vi "EventLog.Gui.vi"() -> ()   [LabVIEW 2016]
uses:
  <vilib>/Utility/miscctls.llb/LVRowAndColumnUnsignedTypeDef.ctl
  EventLog.Buffer.Action.ctl
  Global/ApplicationGlobal.vi
  Config/Config.Global.vi
  Translator/Translator.Global.vi
panel:
  out "error out":errorcluster
  out "Panel":refnum<vi>
  out "_loop":i32(ring)=4
  out "Events":i32(listbox)
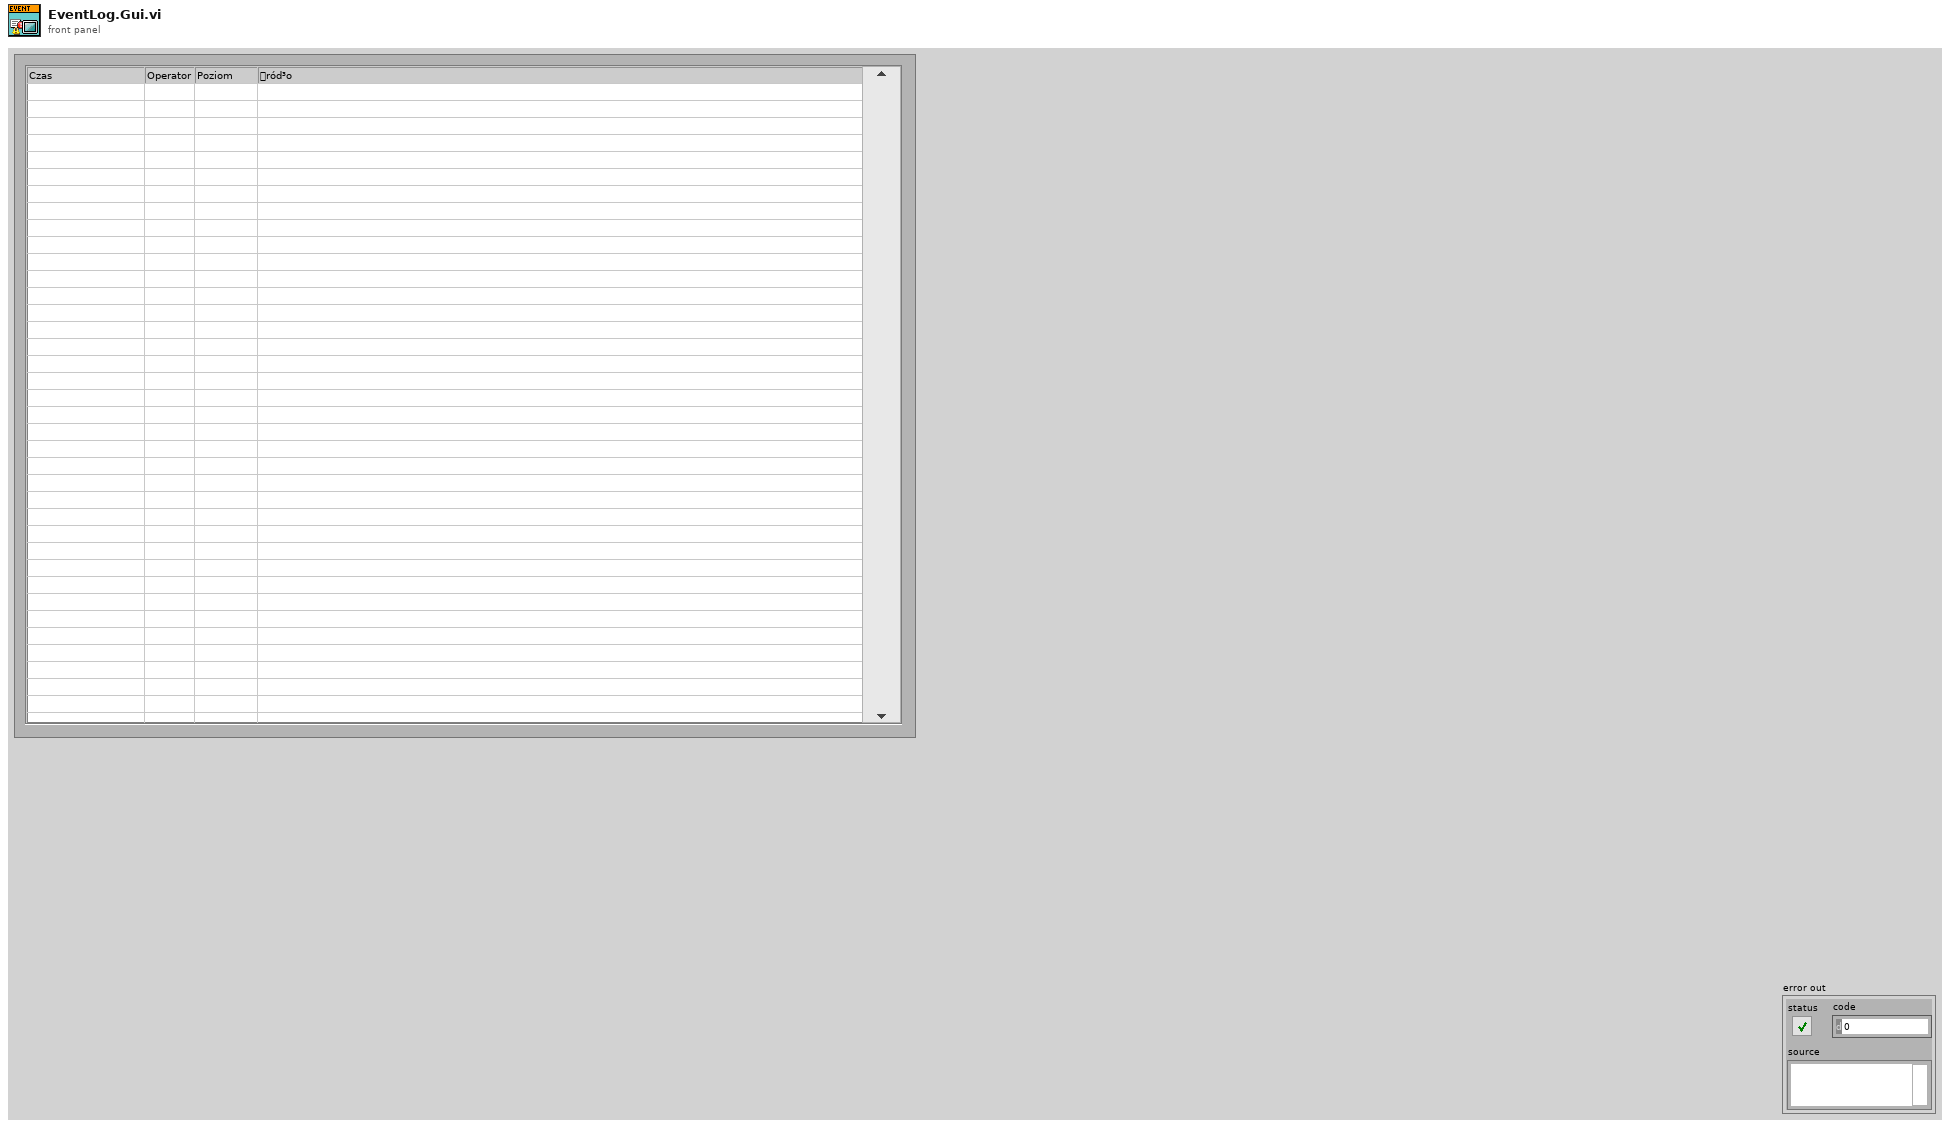
[diagram p1: front panel]
types:
  T1 = typedef "LVRowAndColumnUnsignedTypeDef.ctl" = cluster{"Row":u32, "Column":u32}
  T2 = typedef "EventLog.Buffer.Action.ctl" = enum16{"init", "re-init", "clear", "set translator", "add", "get", "get unsaved"}
  T3 = typedef "LVPositionTypeDef.ctl" = cluster{"Left":i32, "Top":i32}
  T4 = typedef "EventLog.Gui.Sets.ctl" = cluster{"IncludeBegin":bool, "dtm_Begin":timestamp, "IncludeEnd":bool, "dtm_End":timestamp, "Events Level Operator":T5, "Level":u16, "Source":u16, "SearchText":string, "Freeze":bool}
  T5 = typedef "EventLog.EventLevelOperatorGui.ctl" = enum16{">=", "=", "<="}
  T6 = enum32{"Invalid", "Standard", "Closed", "Hidden", "Minimized", "Maximized"}
  T7 = typedef "EventLog.EventGui.ctl" = cluster{"ts":dbl, "lev":T8, "usr":i32, "src":T9, "msg":T10, "arg":variant[], "msg_str":string}
  T8 = typedef "EventLog.EventLevel.ctl" = enum8{"Debug", "Info", "Warning", "Error"}
  T9 = typedef "EventLog.EventSource.ctl" = enum16{"All", "Gui", "Ref", "File", "Arch", "Seq", "CPX", "DB", "Laser", "Scan.P", "Scan.O"}
  T10 = typedef "Translator.Message.ctl" = enum16{"-", "Event confirmed", "Log out", "Log in", "Shutdown", "Cancel", "Start", "Begin time", "End time", "Duration", "Service Mode", "Ignore Results", "Serial Format", "On", "Off", "OK", "NOK", "NOK %s", "Home", "Work", "Close", "Open", "In progress...", "Missing", "Empty", "Hardware failure", "Initial", "Default", "Total", "Out of range", "Free disk space is below 1GB - contact technician", "Error %d >> %s", "Error %d >> %s >> %s", "Msg %d >> %s", "Laser msg %d %s", "Laser cmd error %s %d", "Laser cmd failed %s", "Laser cmd warning %s", "Laser disconnected", "Laser status %s", "Laser already started", "Laser job unkonwn %s", "Laser job missing %s", "Laser job select failure %s", "Unable to start laser printing (%s)", "Unable to stop laser printing (%s)", "Laser marking aborted", "Laser marking timeout", "Unable to reset Laser Interlock (%s)", "Unable to trigger Laser. Laser not ready (%s)", "Laser job '%s' coordinates not configured", "Starting %s", "Quitting %s", "Configured", "Initializing", "Quitting", "Loading", "Loaded %d results", "Loaded %d events", "Running", "Stopped", "Summary", "Laser", "Do you want to continue?", "Do you want to delete the configuration?", "The configuration is being used by an order. Unable to delete!", "Press confirm button", "Station is not based. Do you want to exit?", "Station requires changeover. Do you want to run the test?", "Test options are not set as default. Do you want to continue?", "Formatting of WabcoNo is disabled. Do you want to continue?", "Product not detected. Do you want to continue?", "Product scan failed. Do you want to continue?", "Calibration", "Log out?", "System", "All", "IDLE", "Translating...%s", "Not found", "Alarm %s", "Run", "Skip", "Abort", "Repeat", "Please wait...", "Database disconnected", "Database disconnected - changeover disabled!", "Login to database successful", "Login to database failed: %d; %s", "Unable to check the product status of reference %d - database disconnected", "Unable to set the product status of reference %d - database disconnected", "Variant file backup %s", "Read variant (%s)", "Result", "Station armed!", "Station requires changeover!", "Select reference number...", "EMERGENCY BUTTON - press Control button", "EMERGENCY DOOR - press Control button", "Resetting Emergency...", "Unable to reset safety circuit - Emergency Button pressed", "Unable to reset safety circuit - Emergency Side Door open", "Station not based", "Station based", "Station not empty", "Station basing...", "No order", "Press Start to begin new order", "Scanning new order", "Order NOK. Correct or scan again", "Order OK. Press Accept", "Order ready", "Revolver incorrect", "Fork incorrect", "Revolver missing", "Revolver empty", "Container missing", "Offline results", "Offline statistics", "Updating statistics %.1f %%", "DMC Configurator", "Door open", "Close the front door", "Press start button", "Done. Open the front door", "Running...", "Running...%.1f %%", "Pause %s", "Pause %s. NOK container missing", "Pause %s. OK container missing", "Pause %s. Revolver empty", "Pause %s. Revolver missing", "Pause %s. Revolver incorrect", "Pause %s. Fork missing", "Pause %s. Fork incorrect", "Pause %s. Too many failures", "Pause %s. Unloading failure", "Pause %s. One slot is not working", "Pause %s. Part order is done. Empty OK container", "Pause %s. Unable to move product to slot", "Pause %s. Unable to move back product pusher", "Pause %s. Unable to lift product", "Pause %s. Unable to move back product lifter", "Pause %s. Unable to move product arm to Work", "Pause %s. Unable to move product arm to NOK", "Pause %s. Unable to move product arm to OK", "Pause %s. Unable to unsuck the NOK product", "Pause %s. Unable to drop the NOK product", "Pause %s. Product OK missing", "Pause %s. Unable to unsuck the OK product", "Pause %s. Unable to drop the OK product", "Stopping...", "File '%s' is missing", "File '%s' is broken", "File '%s' is running", "Log file started (%s)", "Log file ended (%s)", "Log file stopped (%s)", "Log file ignored (%s)", "Log file exported (%s)", "Log file export failed (%s)", "Wrong serial number in log file", "Wrong reference number in log file", "Test steps are missing", "%s = %.3f", "Process param '%s' not found in DB", "Process param '%s' wrong order", "Process param '%s' value %.3f out of limits (%.3f; %.3f)", "Step%d param '%s' not found in DB", "Step%d param '%s' wrong order", "Step%d param '%s' value %.3f out of limits (%.3f; %.3f)", "Step%d EV '%s' not found in DB", "Step%d EV '%s' wrong order", "\"%s\" not found in DB", "\"%s\" wrong order", "\"%s\" value %.3f out of limits (%.3f; %.3f)", "\"%s\" not found in software", "Process init (%s)", "Process started", "Process restarted", "Process run", "Process done", "Process done - remove OK container", "Process aborted", "Process aborted at work", "Process aborted at home", "Process error", "Process error at home", "Process error at work", "Process close", "Process pause", "Process continue", "Process door open", "Process door close", "Process pause at slot %s due to %s", "Select plate from the order to process", "Do you want to start the process?", "Do you want to continue the process?", "There is unfinished order. Do you want to put the new order?", "Product %s %d OK", "Product %s %d NOK", "Unable to unload the slot %s. Product missing in the slot", "Unable to unload the slot %s. Product already in the arm", "Unable to accept the product as OK. Product missing in slot %s", "Unable to accept the product as OK. Product could not drop into the container at slot %s", "Unable to accept the product as NOK. Product could not drop into the container at slot %s", "Scan failed. Error %s", "Scan failed. Scanner disconnected", "Scan failed. Wrong Wabco number %d, limit (%d,%d)", "Scan failed. Wrong serial number %d, limit (%d,%d)", "Scan failed. Wrong date %d, limit (%d,%d)", "Scan failed. Wrong product wabco number %d (expected %d)", "Scan failed. Wrong product serial number %d (expected > 0)", "Scan OK %s", "Scan failed. Unable to determine table position (%s)", "Scan failed. Timeout", "Tune failed. Scanner disconnected", "Tune failed. Timeout", "%s = %d", "%s = %d->%d", "Unable to set %s = %.2f - Air Pressure Inside off", "Unable to set digital output '%s' = %d", "Unable to activate air pressure inside - timeout", "Unable to activate air pressure inside - aborted", "Unable to switch on Air Main Valve - Air Pressure Inlet off", "Unable to switch on Air Main Valve - Door open", "Unable to switch off Air Main Valve - timeout", "Unable to switch off Air Main Valve - aborted", "Unable to rotate Table - timeout", "Unable to rotate Table - aborted", "Unable to rotate Table - Product Move not in Home position", "Unable to rotate Table - Air Pressure Inside off", "Unable to rotate Table - Product Lift A not in Home position", "Unable to rotate Table - Product Lift B not in Home position", "Unable to rotate Table - unlock before movement timeout", "Unable to rotate Table - lock after movement timeout", "Unable to move Table Lock to %s position - timeout", "Unable to move Table Lock to %s position - aborted", "Unable to move Table Lock to %s position - Air Pressure Inside off", "Unable to move Table Lock to %s position - Table not in position", "Unable to move Product Lift A to %s position - timeout", "Unable to move Product Lift B to %s position - timeout", "Unable to move Product Lift A to %s position - aborted", "Unable to move Product Lift B to %s position - aborted", "Unable to move Product Lift A to %s position - Air Pressure Inside off", "Unable to move Product Lift B to %s position - Air Pressure Inside off", "Unable to move Product Lift A to %s position - Table not locked", "Unable to move Product Lift B to %s position - Table not locked", "Unable to move Product Lift A to %s position - Product Arm not in Work position", "Unable to move Product Lift B to %s position - Product Arm not in Work position", "Unable to set Product Suction Gripper %s to %s - timeout", "Unable to set Product Suction Gripper %s to %s - aborted", "Unable to set Product Suction Gripper %s to %s - Air Pressure Inside off", "Unable to set Product Suction Gripper %s to %s - Table slot unkown", "Unable to move Product Arm to %s position - timeout", "Unable to move Product Arm to %s position - aborted", "Unable to move Product Arm to %s position - Air Pressure Inside off", "Unable to move Product Arm to %s position - Product Lift A not in Home position", "Unable to move Product Arm to %s position - Product Lift B not in Home position", "Unable to move Product to %s position - timeout", "Unable to move Product to %s position - aborted", "Unable to move Product to %s position - Air Pressure Inside off", "Unable to move Product to %s position - Table not in position"}
  T11 = cluster{"ts":dbl, "lev":T8, "usr":i32, "src":T9, "msg":T10, "arg":variant[]}
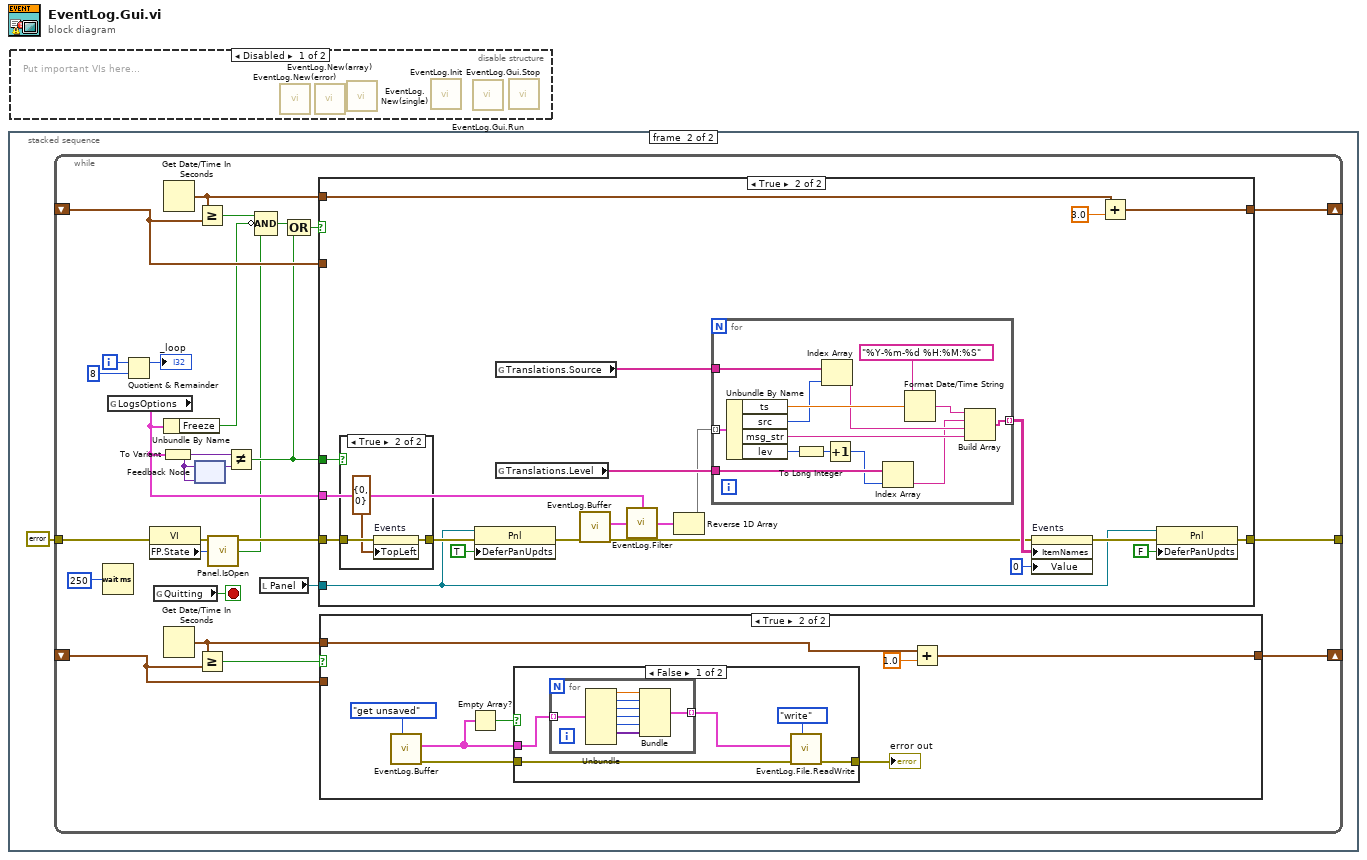
[diagram p0: block diagram]
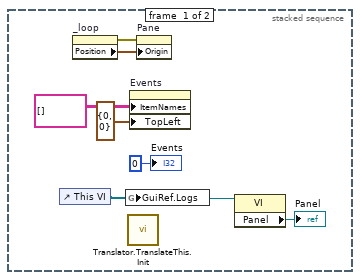
[diagram p2: hidden frame]
diagram:
  n1 = stacked-sequence {
    frame #0 {
      n2 = control-ref of="This VI"() -> (w2:refnum<vi>)
      n3 = property on="_loop" class="Ring (strict)"() -> (error out=w7:errorcluster, "Position"=w6:T3)  [unwired: 2 in, 1 out]
      n4 = global write "ApplicationGlobal.vi" "GuiRef.Logs"(w2) -> ()
      n5 = call "Translator.TranslateThis.Init.vi"() -> ()  [unwired: 11 in, 1 out]
      n6 = property on="Events" class="MCListbox (strict)"("ItemNames"=string[][] [] ("Item Names"), "TopLeft"=T1 {"Row"=0, "Column"=0} ("Top Left Visible Cell")) -> ()  [unwired: 2 in, 2 out]
      n7 = property on="Pane" class="Pane"(error in=w7, "Origin"=w6) -> ()  [unwired: 1 in, 2 out]
      n8 = property class="VI"(reference=w2) -> ("Panel"=→"Panel":refnum<vi>)  [unwired: 1 in, 2 out]
      "Events" <- 0 ("Events")
    }
    frame #1 {
      n9 = while {
        shift-right: [w34] -> _
        shift-left: _ -> [w33]
        tunnel: errorcluster {"status"=FALSE, "code"=0, "source"=""} ("error out") -> [w31]
        tunnel: [w32] -> _
        shift-right: [w13] -> _
        shift-left: _ -> [w11]
        i -> [w17]
        stop <- w29 stop-if-true
        n10 = Wait (ms)(milliseconds to wait=u32 250) -> ()  [unwired: 1 out]
        n11 = global read "Config.Global.vi" "LogsOptions"() -> (w28:T4)
        n12 = Quotient & Remainder(x=w17, y=8) -> (x-y*floor(x/y)=→"_loop":i32)  [unwired: 1 out]
        n13 = property class="VI"(error in=w31) -> (error out=w30:errorcluster, "FP.State"=w10:T6)  [unwired: 1 in, 1 out]
        n14 = global read "ApplicationGlobal.vi" "Quitting"() -> (w29:bool)
        n15 = To Variant(anything=w28) -> (Variant=w23:variant)
        n16 = Get Date/Time In Seconds() -> (seconds since 1Jan1904=w25:timestamp)
        n17 = Unbundle By Name(w28) -> ("Freeze"=w24:bool)
        n18 = Get Date/Time In Seconds() -> (seconds since 1Jan1904=w14:timestamp)
        n19 = feedback #1(w23) -> (w22:variant)
        n20 = feedback-in #1(w23) -> ()
        n21 = Greater Or Equal?(x=w25, y=w33) -> (x >= y?=w27:bool)
        n22 = Greater Or Equal?(x=w14, y=w11) -> (x >= y?=w12:bool)
        n23 = call "Panel.IsOpen.vi"("FP State"=w10) -> ("Open?"=w9:bool)
        n24 = Not Equal?(x=w23, y=w22) -> (x != y?=w20:bool)
        n25 = Compound Arithmetic op=AND(w27, invert w24, w9) -> (w26:bool)
        n26 = local read "Panel"() -> (w15:refnum<vi>)
        n27 = Compound Arithmetic op=OR(w26, w20) -> (w19:bool)
        n28 = case shown="True" w19 {
          tunnel: w30 -> [w59 w72]
          tunnel: [w59 w64] -> w32
          tunnel: [w58 w77] -> w34
          tunnel: w25 -> [_ w76]
          tunnel: w33 -> [w58 _]
          tunnel: w28 -> [_ w60]
          tunnel: w20 -> [_ w71]
          tunnel: w15 -> [_ w66]
          frame False {
          }
          frame True {
            n29 = case shown="True" w71 {
              tunnel: w72 -> [w81 w84]
              tunnel: [w81 w83] -> w69
              frame False {
              }
              frame True {
                n30 = property on="Events" class="MCListbox (strict)"(error in=w84, "TopLeft"=T1 {"Row"=0, "Column"=0} ("Top Left Visible Cell")) -> (error out=w83:errorcluster)  [unwired: 1 in, 1 out]
              }
            }
            n31 = property class="Pnl"(reference=w66, error in=w69, "DeferPanUpdts"=TRUE ("Defer Panel Updates")) -> (error out=w68:errorcluster)  [unwired: 1 out]
            n32 = global read "Translator.Global.vi" "Translations.Source"() -> (w73:string[])
            n33 = global read "Translator.Global.vi" "Translations.Level"() -> (w80:string[])
            n34 = call "EventLog.Buffer.vi"("error in"=w68) -> ("error out"=w78:errorcluster, "data out"=w62:T7[])  [unwired: 7 in, 2 out]
            n35 = call "EventLog.Filter.vi"("data in"=w62, "Event.Sets"=w60) -> ("data out"=w63:T7[])
            n36 = Reverse 1D Array(array=w63) -> (reversed array=w61:T7[])
            n37 = for {
              tunnel: [w96] -> w79 mode=indexing
              tunnel: w61 -> [w95] mode=indexing
              tunnel: w80 -> [w93]
              tunnel: w73 -> [w89]
              n38 = Unbundle By Name(w95) -> ("ts"=w97:dbl, "src"=w87:T9, "msg_str"=w92:string, "lev"=w91:T8)
              n39 = To Long Integer(number=w91) -> (32bit integer=w86:i32)
              n40 = Index Array(array=w89, index=w87) -> (element=w88:string)
              n41 = Increment(x=w86) -> (x+1=w90:i32)
              n42 = Index Array(array=w93, index=w90) -> (element=w85:string)
              n43 = Format Date/Time String(time format string (%c)="%Y-%m-%d %H:%M:%S", seconds (now)=w97) -> (date/time string=w94:string)  [unwired: 1 in]
              n44 = Build Array(w94, w85, w88, w92) -> (w96:string[])
            }
            n45 = property on="Events" class="MCListbox (strict)"(error in=w78, "ItemNames"=w79, "Value"=0 ("Events")) -> (error out=w67:errorcluster)  [unwired: 1 in, 1 out]
            n46 = Add(x=w76, y=3.0) -> (x+y=w77:timestamp)
            n47 = property class="Pnl"(reference=w66, error in=w67, "DeferPanUpdts"=FALSE ("Defer Panel Updates")) -> (error out=w64:errorcluster)  [unwired: 1 out]
          }
        }
        n48 = case shown="True" w12 {
          tunnel: w14 -> [_ w37]
          tunnel: [w35 w36] -> w13
          tunnel: w11 -> [w35 _]
          frame False {
          }
          frame True {
            n49 = call "EventLog.Buffer.vi"("action (get)"=EventLog.Buffer.Action."get unsaved") -> ("error out"=w42:errorcluster, "data out"=w41:T7[])  [unwired: 7 in, 2 out]
            n50 = Empty Array?(array=w41) -> (empty?=w40:bool)
            n51 = case shown="False" w40 {
              tunnel: w42 -> [w47 w57]
              tunnel: w41 -> [w45 _]
              tunnel: [w46 w57] -> w39
              frame False {
                n52 = for {
                  tunnel: w45 -> [w56] mode=indexing
                  tunnel: [w49] -> w44 mode=indexing
                  n53 = Unbundle(w56) -> ("ts"=w55:dbl, "lev"=w54:T8, "usr"=w52:i32, "src"=w53:T9, "msg"=w51:T10, "arg"=w50:variant[])  [unwired: 1 out]
                  n54 = Bundle("ts"=w55, "lev"=w54, "usr"=w52, "src"=w53, "msg"=w51, "arg"=w50) -> (w49:T11)  [unwired: 1 in]
                }
                n55 = call "EventLog.File.ReadWrite.vi"("action (read)"=enum16{"read", "write"}."write", "error in"=w47, "Events in"=w44) -> ("error out"=w46:errorcluster)  [unwired: 4 in, 4 out]
              }
              frame True {
              }
            }
            "error out" <- w39
            n56 = Add(x=w37, y=1.0) -> (x+y=w36:timestamp)
          }
        }
      }
    }
  }
  n57 = disable-structure shown="Disabled" {
    frame Disabled {
      # "Put important VIs here..."
      n58 = call "EventLog.New(error).vi"() -> ()  [unwired: 11 in, 1 out]
      n59 = call "EventLog.New(array).vi"() -> ()  [unwired: 10 in, 2 out]
      n60 = call "EventLog.New(single).vi"() -> ()  [unwired: 10 in, 2 out]
      n61 = call "EventLog.Init.vi"() -> ()  [unwired: 11 in, 1 out]
      n62 = call "EventLog.Gui.Run.vi"() -> ()  [unwired: 10 in, 2 out]
      n63 = call "EventLog.Gui.Stop.vi"() -> ()  [unwired: 11 in, 1 out]
    }
    frame Enabled {
    }
  }
